vi "Send Command Query (non-enum).vi"(8 "error in (no error)":errorcluster, 10 "Command":string, 11 "Gen 2 in":refnum<class "Gen 2.lvclass">) -> (0 "error out":errorcluster, 2 "Response":string, 3 "Gen 2 out":refnum<class "Gen 2.lvclass">)   [LabVIEW 2018, in "Gen 2.lvlib" / "Gen 2.lvclass"]
doc: "This Override is used to send a command to the targeted device and read the reponse\nNOTE: This Override was created to provide means to sends commands that are not part of the Command LIst.ctl whic was initially intended for Model H Laser (Kronos)"
uses:
  Gen 2.lvclass
  PPLs/Laser/Parent/Laser.lvlibp/Laser.lvclass
  C:/Projects/LabVIEW/PPLs/Laser/Parent/Laser.lvlibp/Laser.lvclass
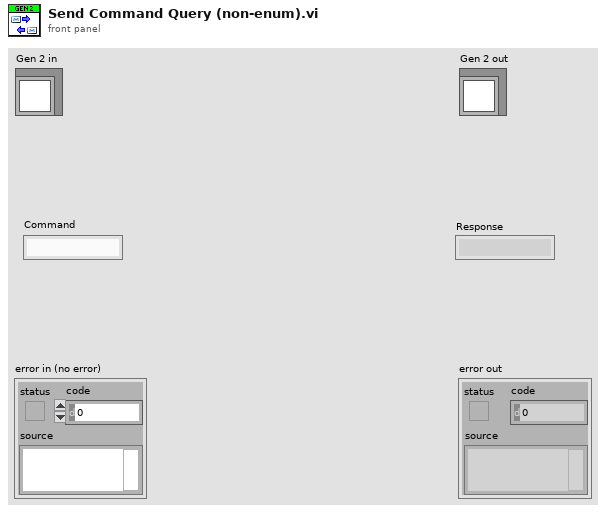
[diagram p1: front panel]
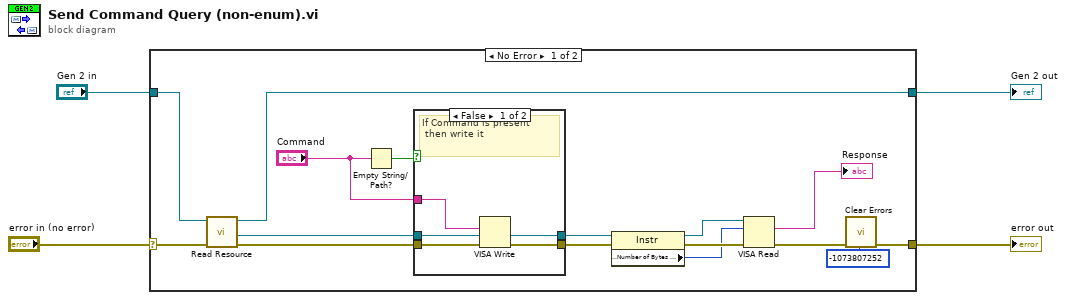
[diagram p0: block diagram]
diagram:
  n1 = case shown="No Error" "error in (no error)" {
    selector: "error in (no error)" -> [w19 w28]
    tunnel: "Gen 2 in" -> [w20 w29]
    tunnel: [w18 w29] -> w2
    tunnel: [w5 w28] -> w1
    frame No Error {
      n2 = call "Read Resource.vi"("error in (no error)"=w19, "Laser in"=w20) -> ("error out"=w17:errorcluster, "Resource"=w16:refnum<visa-resource-name>, "Laser out"=w18:refnum<class "Gen 2.lvclass">)  [unwired: 7 in]
      n3 = Empty String/Path?(string/path="Command") -> (empty?=w11:bool)
      n4 = case shown="False" w11 {
        tunnel: w17 -> [w25 w26]
        tunnel: w16 -> [w24 w27]
        tunnel: [w23 w26] -> w9
        tunnel: [w22 w27] -> w10
        tunnel: "Command" -> [w21 _]
        frame False {
          # "If Command is present\n then write it"
          n5 = VISA Write(VISA resource name=w24, write buffer=w21, error in (no error)=w25) -> (VISA resource name out=w22:refnum<visa-resource-name>, error out=w23:errorcluster)  [unwired: 1 out]
        }
        frame True {
          # "Empty Command asks as a\nport listener for the class"
        }
      }
      n6 = property class="Instr"(reference=w10, error in=w9) -> (reference out=w14:refnum<visa-resource-name>, error out=w15:errorcluster, "Serial Settings:Number of Bytes at Serial Port"=w8:u32)
      n7 = VISA Read(VISA resource name=w14, byte count=w8, error in (no error)=w15) -> (read buffer=→"Response":string, error out=w7:errorcluster)  [unwired: 2 out]
      n8 = call <vilib>:"Clear Errors.vi"("error in (no error)"=w7, "specific error code to clear (0: all)"=-1073807252) -> ("error out"=w5:errorcluster)  [unwired: 4 in, 1 out]
    }
    frame Error {
    }
  }
  "error out" <- w1
  "Gen 2 out" <- w2
